vi "FPGA Accumulate Coil Volts.vi"(11 "Data Array In":T1=[0, 0, 0, 0, 0, 0, 0, 0, 0, 0, 0, 0, 0, 0, 0, 0, 0, 0, 0, 0, 0, 0, 0, 0, 0, 0, 0, 0, 0, 0, 0, 0, 0, 0, 0, 0, 0, 0]) -> (3 "Data Array Out":T1)   [LabVIEW 2018]
doc: "Author: Scott Hannahs <sth@magnet.fsu.edu>\nCopyright 2018 Florida State University, All rights reserved."
uses:
  <vilib>/eio/EIONode/EIONode.xnode
  <vilib>/rvi/eio/common/nirviEmuTemplateMethod_errors.vi
  SCH Data Controls/SCH Raw Int Data.ctl
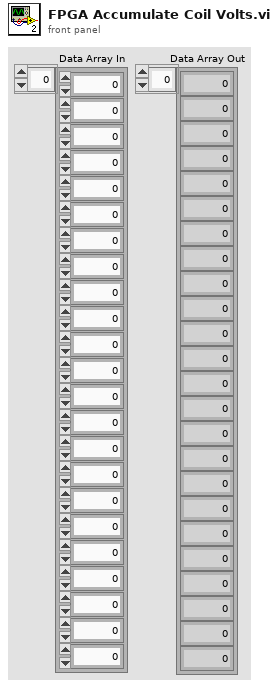
[diagram p1: front panel]
types:
  T1 = typedef "SCH Raw Int Data.ctl" = i16[]
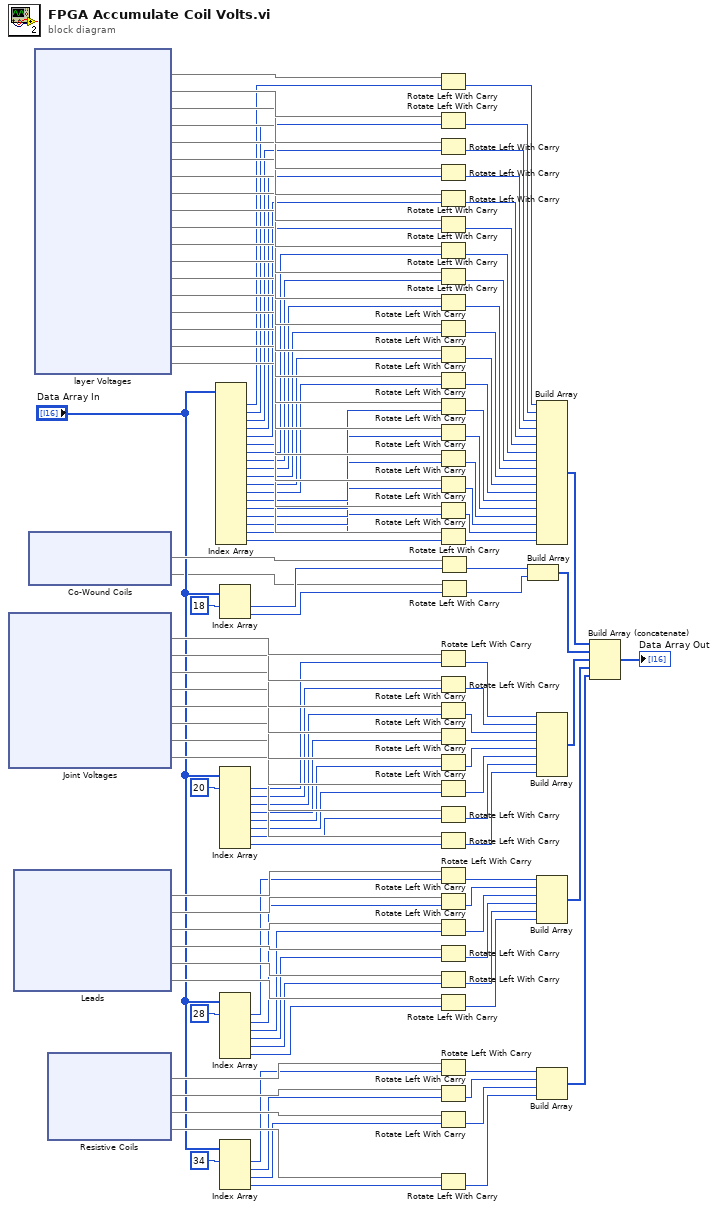
[diagram p0: block diagram]
diagram:
  n1 = xnode "Joint Voltages"() -> ("Cold Mass Inlet Joint"=w107, "Cold Mass Outlet Joint"=w106, "Inlet Lead 4K Joint"=w105, "Outlet Lead 4K Joint"=w104, "HF-MF Joint"=w103, "MF-LF1 Joint"=w102, "LF1-LF2 Joint"=w101, "LF2-LF3 Joint"=w100)  [unwired: 8 in, 8 out]
  n2 = xnode "Leads"() -> ("Inlet Lead RT-77K"=w98, "Outlet Lead RT to 77K"=w97, "Inlet Lead 77K-4K"=w96, "Outlet Lead 77K to 4K"=w95, "Inlet SC Bus"=w94, "Outlet SC Bus"=w93)  [unwired: 6 in, 6 out]
  n3 = xnode "Co-Wound Coils"() -> ("Co-Wound Coil #1"=w99, "Dump Resistor"=w5)  [unwired: 2 in, 2 out]
  n4 = xnode "layer Voltages"() -> ("Layer #1 Voltage"=w109, "Layer #2 Voltage"=w125, "Layer #3 Voltage"=w124, "Layer #4 Voltage"=w123, "Layer #5 Voltage"=w122, "Layer #6 Voltage"=w121, "Layer #7 Voltage"=w120, "Layer #8 Voltage"=w119, "Layer #9 Voltage"=w118, "Layer #10 Voltage"=w117, "Layer #11 Voltage"=w116, "Layer #12 Voltage"=w115, "Layer #13 Voltage"=w114, "Layer #14 Voltage"=w113, "Layer #15 Voltage"=w112, "Layer #16 Voltage"=w111, "Layer #17 Voltage"=w110, "Layer #18 Voltage"=w108)  [unwired: 18 in, 18 out]
  n5 = xnode "Resistive Coils"() -> ("Resistive Coil A"=w92, "Resistive Coil B"=w91, "Resistive Coil C"=w90, "Resistive Coil D"=w89)  [unwired: 4 in, 4 out]
  n6 = Index Array(array="Data Array In") -> (element #1=w83:i16, element #2=w82:i16, element #3=w81:i16, element #4=w80:i16, element #5=w79:i16, element #6=w78:i16, element #7=w77:i16, element #8=w76:i16, element #9=w75:i16, element #10=w74:i16, element #11=w73:i16, element #12=w72:i16, element #13=w71:i16, element #14=w70:i16, element #15=w69:i16, element #16=w51:i16, element #17=w50:i16, element #18=w48:i16)  [unwired: 18 in]
  n7 = Index Array(array="Data Array In", index #1=18 ("index")) -> (element #1=w29:i16, element #2=w4:i16)  [unwired: 1 in]
  n8 = Index Array(array="Data Array In", index #1=20 ("index")) -> (element #1=w46:i16, element #2=w45:i16, element #3=w44:i16, element #4=w43:i16, element #5=w42:i16, element #6=w41:i16, element #7=w40:i16, element #8=w39:i16)  [unwired: 7 in]
  n9 = Index Array(array="Data Array In", index #1=28 ("index")) -> (element #1=w16:i16, element #2=w17:i16, element #3=w25:i16, element #4=w26:i16, element #5=w27:i16, element #6=w28:i16)  [unwired: 5 in]
  n10 = Index Array(array="Data Array In", index #1=34 ("index")) -> (element #1=w15:i16, element #2=w14:i16, element #3=w8:i16, element #4=w7:i16)  [unwired: 3 in]
  n11 = Rotate Left With Carry(2:w83, 3:w109) -> (0:w68:i16)  [unwired: 1 out]
  n12 = Rotate Left With Carry(2:w82, 3:w125) -> (0:w67:i16)  [unwired: 1 out]
  n13 = Rotate Left With Carry(2:w81, 3:w124) -> (0:w66:i16)  [unwired: 1 out]
  n14 = Rotate Left With Carry(2:w80, 3:w123) -> (0:w65:i16)  [unwired: 1 out]
  n15 = Rotate Left With Carry(2:w79, 3:w122) -> (0:w64:i16)  [unwired: 1 out]
  n16 = Rotate Left With Carry(2:w78, 3:w121) -> (0:w63:i16)  [unwired: 1 out]
  n17 = Rotate Left With Carry(2:w77, 3:w120) -> (0:w62:i16)  [unwired: 1 out]
  n18 = Rotate Left With Carry(2:w76, 3:w119) -> (0:w61:i16)  [unwired: 1 out]
  n19 = Rotate Left With Carry(2:w75, 3:w118) -> (0:w60:i16)  [unwired: 1 out]
  n20 = Rotate Left With Carry(2:w74, 3:w117) -> (0:w59:i16)  [unwired: 1 out]
  n21 = Rotate Left With Carry(2:w73, 3:w116) -> (0:w58:i16)  [unwired: 1 out]
  n22 = Rotate Left With Carry(2:w72, 3:w115) -> (0:w57:i16)  [unwired: 1 out]
  n23 = Rotate Left With Carry(2:w71, 3:w114) -> (0:w56:i16)  [unwired: 1 out]
  n24 = Rotate Left With Carry(2:w70, 3:w113) -> (0:w55:i16)  [unwired: 1 out]
  n25 = Rotate Left With Carry(2:w69, 3:w112) -> (0:w54:i16)  [unwired: 1 out]
  n26 = Rotate Left With Carry(2:w51, 3:w111) -> (0:w53:i16)  [unwired: 1 out]
  n27 = Rotate Left With Carry(2:w50, 3:w110) -> (0:w52:i16)  [unwired: 1 out]
  n28 = Rotate Left With Carry(2:w48, 3:w108) -> (0:w49:i16)  [unwired: 1 out]
  n29 = Rotate Left With Carry(2:w46, 3:w107) -> (0:w38:i16)  [unwired: 1 out]
  n30 = Rotate Left With Carry(2:w45, 3:w106) -> (0:w37:i16)  [unwired: 1 out]
  n31 = Rotate Left With Carry(2:w44, 3:w105) -> (0:w36:i16)  [unwired: 1 out]
  n32 = Rotate Left With Carry(2:w43, 3:w104) -> (0:w35:i16)  [unwired: 1 out]
  n33 = Rotate Left With Carry(2:w42, 3:w103) -> (0:w34:i16)  [unwired: 1 out]
  n34 = Rotate Left With Carry(2:w41, 3:w102) -> (0:w33:i16)  [unwired: 1 out]
  n35 = Rotate Left With Carry(2:w40, 3:w101) -> (0:w32:i16)  [unwired: 1 out]
  n36 = Rotate Left With Carry(2:w39, 3:w100) -> (0:w31:i16)  [unwired: 1 out]
  n37 = Rotate Left With Carry(2:w16, 3:w98) -> (0:w19:i16)  [unwired: 1 out]
  n38 = Rotate Left With Carry(2:w17, 3:w97) -> (0:w18:i16)  [unwired: 1 out]
  n39 = Rotate Left With Carry(2:w25, 3:w96) -> (0:w21:i16)  [unwired: 1 out]
  n40 = Rotate Left With Carry(2:w26, 3:w95) -> (0:w22:i16)  [unwired: 1 out]
  n41 = Rotate Left With Carry(2:w27, 3:w94) -> (0:w23:i16)  [unwired: 1 out]
  n42 = Rotate Left With Carry(2:w28, 3:w93) -> (0:w24:i16)  [unwired: 1 out]
  n43 = Rotate Left With Carry(2:w15, 3:w92) -> (0:w12:i16)  [unwired: 1 out]
  n44 = Rotate Left With Carry(2:w14, 3:w91) -> (0:w13:i16)  [unwired: 1 out]
  n45 = Rotate Left With Carry(2:w8, 3:w90) -> (0:w10:i16)  [unwired: 1 out]
  n46 = Rotate Left With Carry(2:w7, 3:w89) -> (0:w9:i16)  [unwired: 1 out]
  n47 = Rotate Left With Carry(2:w29, 3:w99) -> (0:w86:i16)  [unwired: 1 out]
  n48 = Rotate Left With Carry(2:w4, 3:w5) -> (0:w3:i16)  [unwired: 1 out]
  n49 = Build Array(w86, w3) -> (w2:i16[])
  n50 = Build Array(w68, w67, w66, w65, w64, w63, w62, w61, w60, w59, w58, w57, w56, w55, w54, w53, w52, w49) -> (w88:i16[])
  n51 = Build Array(w38, w37, w36, w35, w34, w33, w32, w31) -> (w1:i16[])
  n52 = Build Array(w19, w18, w21, w22, w23, w24) -> (w85:i16[])
  n53 = Build Array(w12, w13, w10, w9) -> (w84:i16[])
  n54 = Build Array (concatenate)(w88, w2, w1, w85, w84) -> (→"Data Array Out":i16[])
